vi "Initialize-object.vi"(8 "error in (no error)":errorcluster, 10 "Settings":T1) -> (0 "error out":errorcluster, 3 "Reference out":T3)   [LabVIEW 2013, in "Server.lvlib" / "Server.lvclass"]
uses:
  Server.lvclass
  Object-reference.ctl
  Settings.ctl
  Supported-module-types.ctl
  Server.lvclass/Server.ctl
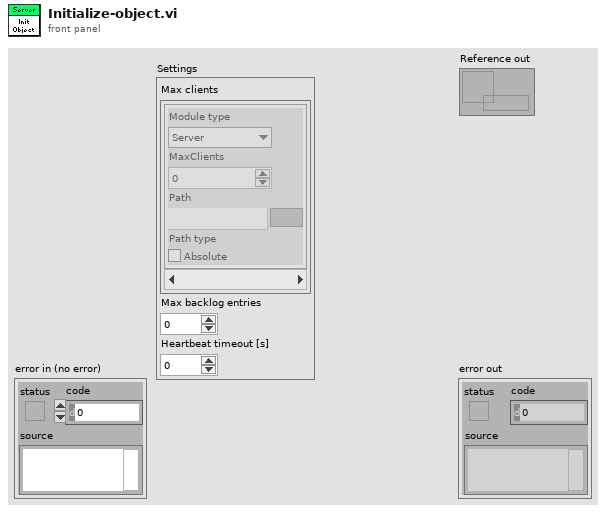
[diagram p1: front panel]
types:
  T1 = typedef "Server.lvlib/Server.lvclass/Settings.ctl" = cluster{"Max clients":cluster{"Module type":T2, "MaxClients":i32, "Path":path, "Path type":bool}[], "Max backlog entries":i32, "Heartbeat timeout":dbl}
  T2 = typedef "Server.lvlib/Server.lvclass/Supported-module-types.ctl" = enum16{"Server", "All", "BeamControl", "PowderDeposition", "StrategyParser", "CameraVision", "MaterialCharacterization", "StatusMonitor", "SLMSimulation", "LaserCharacterization"}
  T3 = typedef "Server.lvlib/Server.lvclass/Object-reference.ctl" = refnum<data-value>
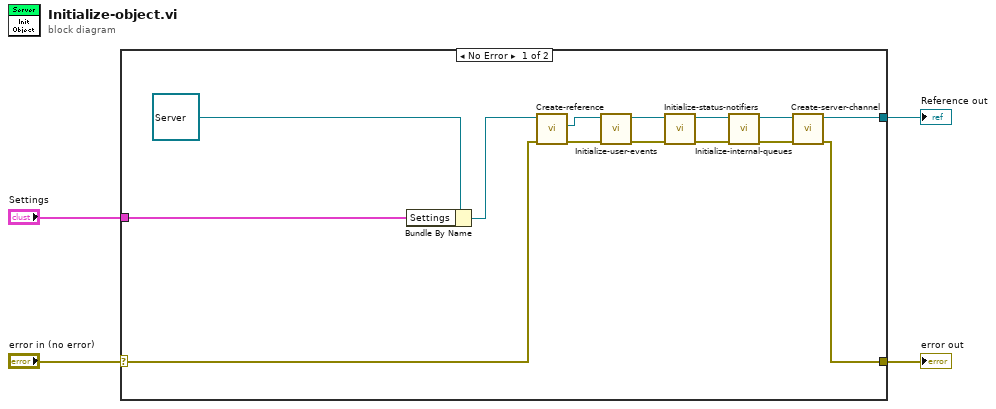
[diagram p0: block diagram]
diagram:
  n1 = case shown="No Error" "error in (no error)" {
    selector: "error in (no error)" -> [w18 w19]
    tunnel: [w5 w19] -> w3
    tunnel: [w6 _] -> w2
    tunnel: "Settings" -> [w15 _]
    frame No Error {
      n2 = Bundle By Name(cluster=refnum<class "Server.lvclass"> refnum ("Panes.lvclass"), "Settings"=w15) -> (w16:refnum<class "Server.lvclass">)
      n3 = call "Create-reference.vi"("error in (no error)"=w18, "Object in"=w16) -> ("error out"=w13:errorcluster, "Object reference"=w14:T3)  [unwired: 7 in, 1 out]
      n4 = call "Initialize-user-events.vi"("error in (no error)"=w13, "ModComm in"=w14) -> ("error out"=w11:errorcluster, "ModComm out"=w12:T3)  [unwired: 8 in]
      n5 = call "Initialize-status-notifiers.vi"("error in (no error)"=w11, "ModComm in"=w12) -> ("error out"=w9:errorcluster, "ModComm out"=w10:T3)  [unwired: 8 in]
      n6 = call "Initialize-internal-queues.vi"("error in (no error)"=w9, "ModComm in"=w10) -> ("error out"=w7:errorcluster, "ModComm out"=w8:T3)  [unwired: 8 in]
      n7 = call "Create-server-channel.vi"("error in (no error)"=w7, "ModComm in"=w8) -> ("error out"=w5:errorcluster, "ModComm out"=w6:T3)  [unwired: 7 in, 1 out]
    }
    frame Error {
    }
  }
  "error out" <- w3
  "Reference out" <- w2
